vi "Plotter.vi"() -> ()   [LabVIEW 2014]
panel:
  in  "Play Button":bool
  in  "Process Stop Button":bool
  in  "Graph 4":u16(ring) items=["---"=0, "REVCNT"=28, "RPM"=1, "TPS"=2, "Air Box Pressure"=3, "H20 Temperature"=4, "Air Temperature"=5, "Oil Temperature"=6, "Battery Voltage"=7, "Oil Pressure"=8, "Lambda 1 Avg."=9, "Lambda 1 Raw"=10, "Lambda 2 Avg."=11, "Lambda 2 Raw"=12, "K Lambda 1"=13, "K Lambda 2"=14, "Inj Low"=15, "Spark"=16, "Phase Low"=17, "Phase High"=18, "Speed"=19, "DTPS+"=20, "DTPS-"=21, "DECA*1"=22, "DECA*2"=23, "Potentiometer Front Left"=24, "Potentiometer Front Right"=25, "Potentiometer Rear Left"=26, "Potentiometer Rear Right"=27, "Gear"=29]
  in  "Graph 3":u16(ring) items=["---"=0, "REVCNT"=28, "RPM"=1, "TPS"=2, "Air Box Pressure"=3, "H20 Temperature"=4, "Air Temperature"=5, "Oil Temperature"=6, "Battery Voltage"=7, "Oil Pressure"=8, "Lambda 1 Avg."=9, "Lambda 1 Raw"=10, "Lambda 2 Avg."=11, "Lambda 2 Raw"=12, "K Lambda 1"=13, "K Lambda 2"=14, "Inj Low"=15, "Spark"=16, "Phase Low"=17, "Phase High"=18, "Speed"=19, "DTPS+"=20, "DTPS-"=21, "DECA*1"=22, "DECA*2"=23, "Potentiometer Front Left"=24, "Potentiometer Front Right"=25, "Potentiometer Rear Left"=26, "Potentiometer Rear Right"=27, "Gear"=29]
  in  "Graph 2":u16(ring) items=["---"=0, "REVCNT"=28, "RPM"=1, "TPS"=2, "Air Box Pressure"=3, "H20 Temperature"=4, "Air Temperature"=5, "Oil Temperature"=6, "Battery Voltage"=7, "Oil Pressure"=8, "Lambda 1 Avg."=9, "Lambda 1 Raw"=10, "Lambda 2 Avg."=11, "Lambda 2 Raw"=12, "K Lambda 1"=13, "K Lambda 2"=14, "Inj Low"=15, "Spark"=16, "Phase Low"=17, "Phase High"=18, "Speed"=19, "DTPS+"=20, "DTPS-"=21, "DECA*1"=22, "DECA*2"=23, "Potentiometer Front Left"=24, "Potentiometer Front Right"=25, "Potentiometer Rear Left"=26, "Potentiometer Rear Right"=27, "Gear"=29]
  out "4":cluster{"Time":dbl[], "Vbb2":dbl[]}(graph)
  out "3":cluster{"Time":dbl[], "Vbb2":dbl[]}(graph)
  in  "Graph 1":u16(ring) items=["---"=0, "REVCNT"=28, "RPM"=1, "TPS"=2, "Air Box Pressure"=3, "H20 Temperature"=4, "Air Temperature"=5, "Oil Temperature"=6, "Battery Voltage"=7, "Oil Pressure"=8, "Lambda 1 Avg."=9, "Lambda 1 Raw"=10, "Lambda 2 Avg."=11, "Lambda 2 Raw"=12, "K Lambda 1"=13, "K Lambda 2"=14, "Inj Low"=15, "Spark"=16, "Phase Low"=17, "Phase High"=18, "Speed"=19, "DTPS+"=20, "DTPS-"=21, "DECA*1"=22, "DECA*2"=23, "Potentiometer Front Left"=24, "Potentiometer Front Right"=25, "Potentiometer Rear Left"=26, "Potentiometer Rear Right"=27, "Gear"=29]
  out "2":cluster{"Time":dbl[], "Vbb2":dbl[]}(graph)
  out "1":cluster{"Time":dbl[], "Vbb2":dbl[]}(graph)
  in  "File path":path
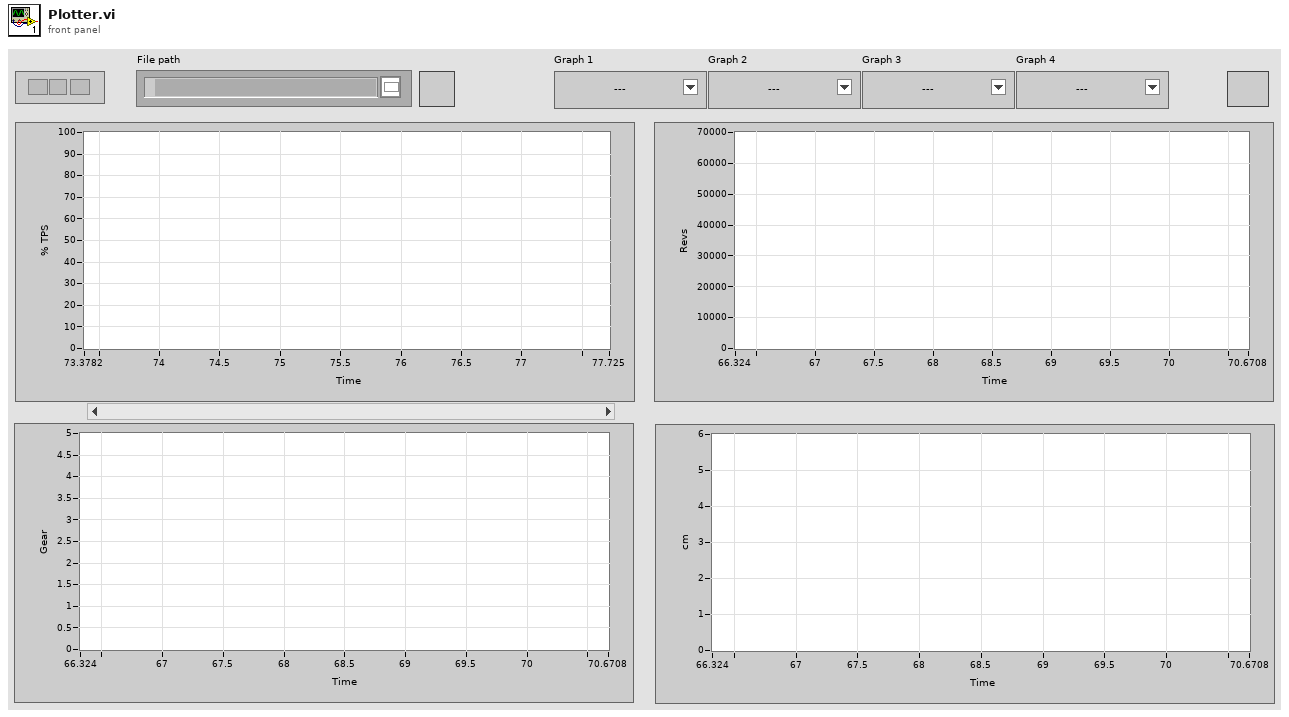
[diagram p1: front panel]
types:
  T1 = typedef "LVRangeTypeDef.ctl" = cluster{"Minimum":dbl, "Maximum":dbl, "Increment":dbl, "Minor Increment":dbl, "Start":dbl}
  T2 = typedef "CAR Data Cluster.ctl" = cluster{"revs":dbl[], "rev/min":dbl[], "TPS":dbl[], "map":dbl[], "T H20":dbl[], "T Air":dbl[], "T Oil":dbl[], "Vbb1":dbl[], "Vbb2":dbl[], "Vbb3":dbl[], "Bar0":dbl[], "Lambda 1 AVG":dbl[], "Lambda 1 RAW":dbl[], "Lambda 2 AVG":dbl[], "Lambda 2 RAW":dbl[], "KLambda 1":dbl[], "KLambda 2":dbl[], "Inj Low":dbl[], "Spark 1":dbl[], "Phase Low":dbl[], "Phase High":dbl[], "Speed 1":dbl[], "Speed 2":dbl[], "DTPS+":dbl[], "DTPS-":dbl[], "DECAYINJ(+) - DECAYINJ(-)":dbl[], "DECAYIGN(+) - DECAYIGN(-)":dbl[], "Pot FL":dbl[], "Pot FR":dbl[], "Pot RL":dbl[], "Pot RR":dbl[], "Time":dbl[]}
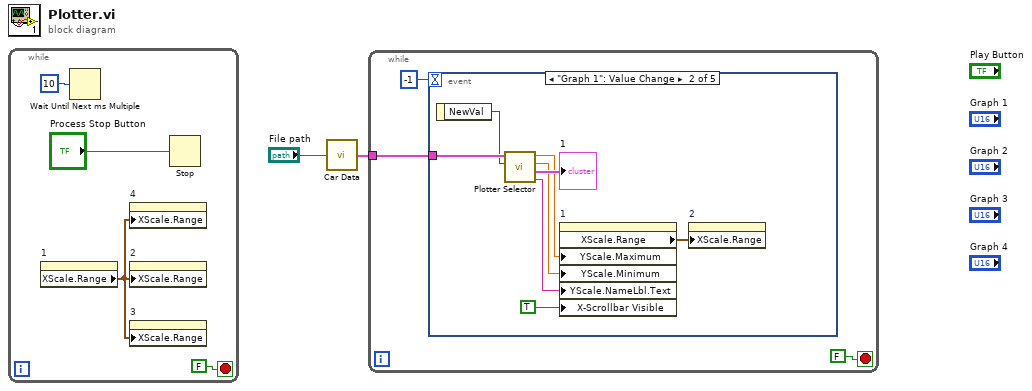
[diagram p0: block diagram]
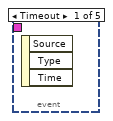
[diagram p2: hidden frame]
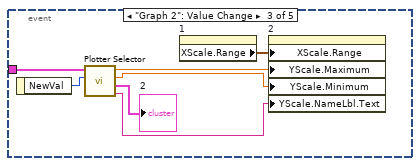
[diagram p3: hidden frame]
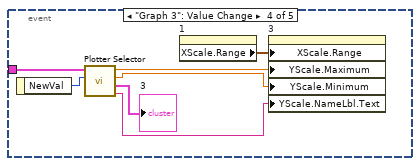
[diagram p4: hidden frame]
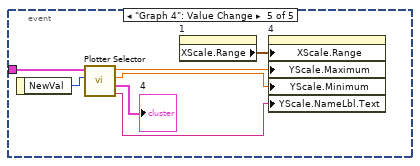
[diagram p5: hidden frame]
diagram:
  n1 = while {
    stop <- FALSE stop-if-true
    n2 = property on="1" class="XYGraph (strict)"() -> ("XScale.Range"=w5:T1)  [unwired: 2 in, 2 out]
    n3 = Wait Until Next ms Multiple(millisecond multiple=u32 10) -> ()  [unwired: 1 out]
    n4 = property on="4" class="XYGraph (strict)"("XScale.Range"=w5) -> ()  [unwired: 2 in, 2 out]
    n5 = property on="2" class="XYGraph (strict)"("XScale.Range"=w5) -> ()  [unwired: 2 in, 2 out]
    n6 = property on="3" class="XYGraph (strict)"("XScale.Range"=w5) -> ()  [unwired: 2 in, 2 out]
    n7 = Stop(stop? (T)="Process Stop Button") -> ()
  }
  n8 = call "Car Data.vi"("file path (dialog if empty)"="File path") -> ("CAR DATA"=w1:T2)
  n9 = while {
    tunnel: w1 -> [w8]
    stop <- FALSE stop-if-true
    n10 = event shown="[1] \"Graph 1\": Value Change" {
      selector: _ -> [_ _ _ _ _]
      dyn-events: _ -> [_ _ _ _ _]
      timeout: -1 -> [_ _ _ _ _]
      tunnel: w8 -> [_ w17 w24 w26 w33]
      event Timeout {
        n11 = event-data() -> ()  [unwired: 1 in, 3 out]
      }
      event "Graph 1": Value Change {
        n12 = event-data() -> ("NewVal"=w16:u16)  [unwired: 1 in]
        n13 = call "Plotter Selector.vi"("Ring Selector"=w16, "CAR DATA"=w17) -> ("Y Label"=w11:string, "Plot Output"=→"1":cluster{"Time":dbl[], "yi":dbl[]}, "Y Minimum"=w12:dbl, "Y Maximum"=w13:dbl)  [unwired: 6 in]
        n14 = property on="1" class="XYGraph (strict)"("YScale.Maximum"=w13, "YScale.Minimum"=w12, "YScale.NameLbl.Text"=w11, "X-Scrollbar Visible"=TRUE ("X Scrollbar Visible")) -> ("XScale.Range"=w14:T1)  [unwired: 2 in, 2 out]
        n15 = property on="2" class="XYGraph (strict)"("XScale.Range"=w14) -> ()  [unwired: 2 in, 2 out]
      }
      event "Graph 2": Value Change {
        n16 = event-data() -> ("NewVal"=w23:u16)  [unwired: 1 in]
        n17 = call "Plotter Selector.vi"("Ring Selector"=w23, "CAR DATA"=w24) -> ("Y Label"=w20:string, "Plot Output"=→"2":cluster{"Time":dbl[], "yi":dbl[]}, "Y Minimum"=w18:dbl, "Y Maximum"=w19:dbl)  [unwired: 6 in]
        n18 = property on="1" class="XYGraph (strict)"() -> ("XScale.Range"=w21:T1)  [unwired: 2 in, 2 out]
        n19 = property on="2" class="XYGraph (strict)"("XScale.Range"=w21, "YScale.Maximum"=w19, "YScale.Minimum"=w18, "YScale.NameLbl.Text"=w20) -> ()  [unwired: 2 in, 2 out]
      }
      event "Graph 3": Value Change {
        n20 = event-data() -> ("NewVal"=w25:u16)  [unwired: 1 in]
        n21 = call "Plotter Selector.vi"("Ring Selector"=w25, "CAR DATA"=w26) -> ("Y Label"=w29:string, "Plot Output"=→"3":cluster{"Time":dbl[], "yi":dbl[]}, "Y Minimum"=w27:dbl, "Y Maximum"=w28:dbl)  [unwired: 6 in]
        n22 = property on="1" class="XYGraph (strict)"() -> ("XScale.Range"=w30:T1)  [unwired: 2 in, 2 out]
        n23 = property on="3" class="XYGraph (strict)"("XScale.Range"=w30, "YScale.Maximum"=w28, "YScale.Minimum"=w27, "YScale.NameLbl.Text"=w29) -> ()  [unwired: 2 in, 2 out]
      }
      event "Graph 4": Value Change {
        n24 = event-data() -> ("NewVal"=w32:u16)  [unwired: 1 in]
        n25 = call "Plotter Selector.vi"("Ring Selector"=w32, "CAR DATA"=w33) -> ("Y Label"=w36:string, "Plot Output"=→"4":cluster{"Time":dbl[], "yi":dbl[]}, "Y Minimum"=w34:dbl, "Y Maximum"=w35:dbl)  [unwired: 6 in]
        n26 = property on="1" class="XYGraph (strict)"() -> ("XScale.Range"=w37:T1)  [unwired: 2 in, 2 out]
        n27 = property on="4" class="XYGraph (strict)"("XScale.Range"=w37, "YScale.Maximum"=w35, "YScale.Minimum"=w34, "YScale.NameLbl.Text"=w36) -> ()  [unwired: 2 in, 2 out]
      }
    }
  }
